vi "host.vi"() -> ()   [LabVIEW 2020]
uses:
  <vilib>/rvi/interface/RandomDataEmulation/nirviRandomDataOpen.vi
  <vilib>/rvi/interface/common/niFpgaCacheSessionInfoDynamic.vi
  <vilib>/Utility/error.llb/Error Cluster From Error Code.vi
  <vilib>/rvi/interface/common/niFpgaWaitOnOcc.vi
  <vilib>/rvi/errors/niLvFpgaAdjustHostInterfaceError.vi
  <vilib>/FPGAPlugInAG/Dynamic/niLvFpga_Run_Dynamic.vi
  <vilib>/FPGAPlugInAG/Dynamic/niLvFpga_Close_Dynamic.vi
  <vilib>/rvi/interface/nirviOpenFPGA/nirviOpenFPGA.xnode
  FFT.vi
  <vilib>/rvi/interface/nirviMethod/nirviMethod.xnode
  <vilib>/rvi/interface/nirviCloseFPGA/nirviCloseFPGA.xnode
  <vilib>/rvi/errors/niLvFpgaMergeErrorWithErrorCode.vi
  <vilib>/FPGAPlugInAG/Dynamic/niLvFpga_ReadFifo_Dynamic.vi
  <vilib>/Analysis/NI_AALPro.lvlib
  <vilib>/FPGAPlugInAG/Dynamic/niLvFpga_ConfigureFifo_Dynamic.vi
  <vilib>/FPGAPlugInAG/Dynamic/niLvFpga_StartFifo_Dynamic.vi
  <vilib>/FPGAPlugInAG/Dynamic/niLvFpga_WriteFifo_Dynamic.vi
panel:
  out "phase 2 index":dbl[](graph)
  out "phase 2 size":i32
  out "mag 2 index":dbl[](graph)
  out "mag 2 size":i32
  out "phase 2":fxp<+/-,32,15>[](array[numeric])
  out "mag 2":fxp<+/-,32,15>[](array[numeric])
  out "frequency index":dbl[](graph)
  out "frequency size":i32
  out "freq":fxp<+/-,32,15>[](array[numeric])
  out "magnitude":dbl[](graph)
  out "phase":dbl[](graph)
  out "phase size":i32
  out "mag size":i32
  out "phase":fxp<+/-,32,15>[](array[numeric])
  out "magnitude":fxp<+/-,32,15>[](array[numeric])
  out "Actual Depth":u32
  out "host to target":u32
  out "signal_target_to_host_fixed size(s)":i32
  out "target to host 1":u32
  out "signal target to host":dbl[][](graph)
  out "signal_target_to_host_fixed":fxp<+/-,24,7>[](array[numeric])
  out "Array 2":fxp<+/-,24,7>[](array[numeric])
  out "detrend acc":dbl[](graph)
  out "samples":i32
  out "input signal":T1(graph)
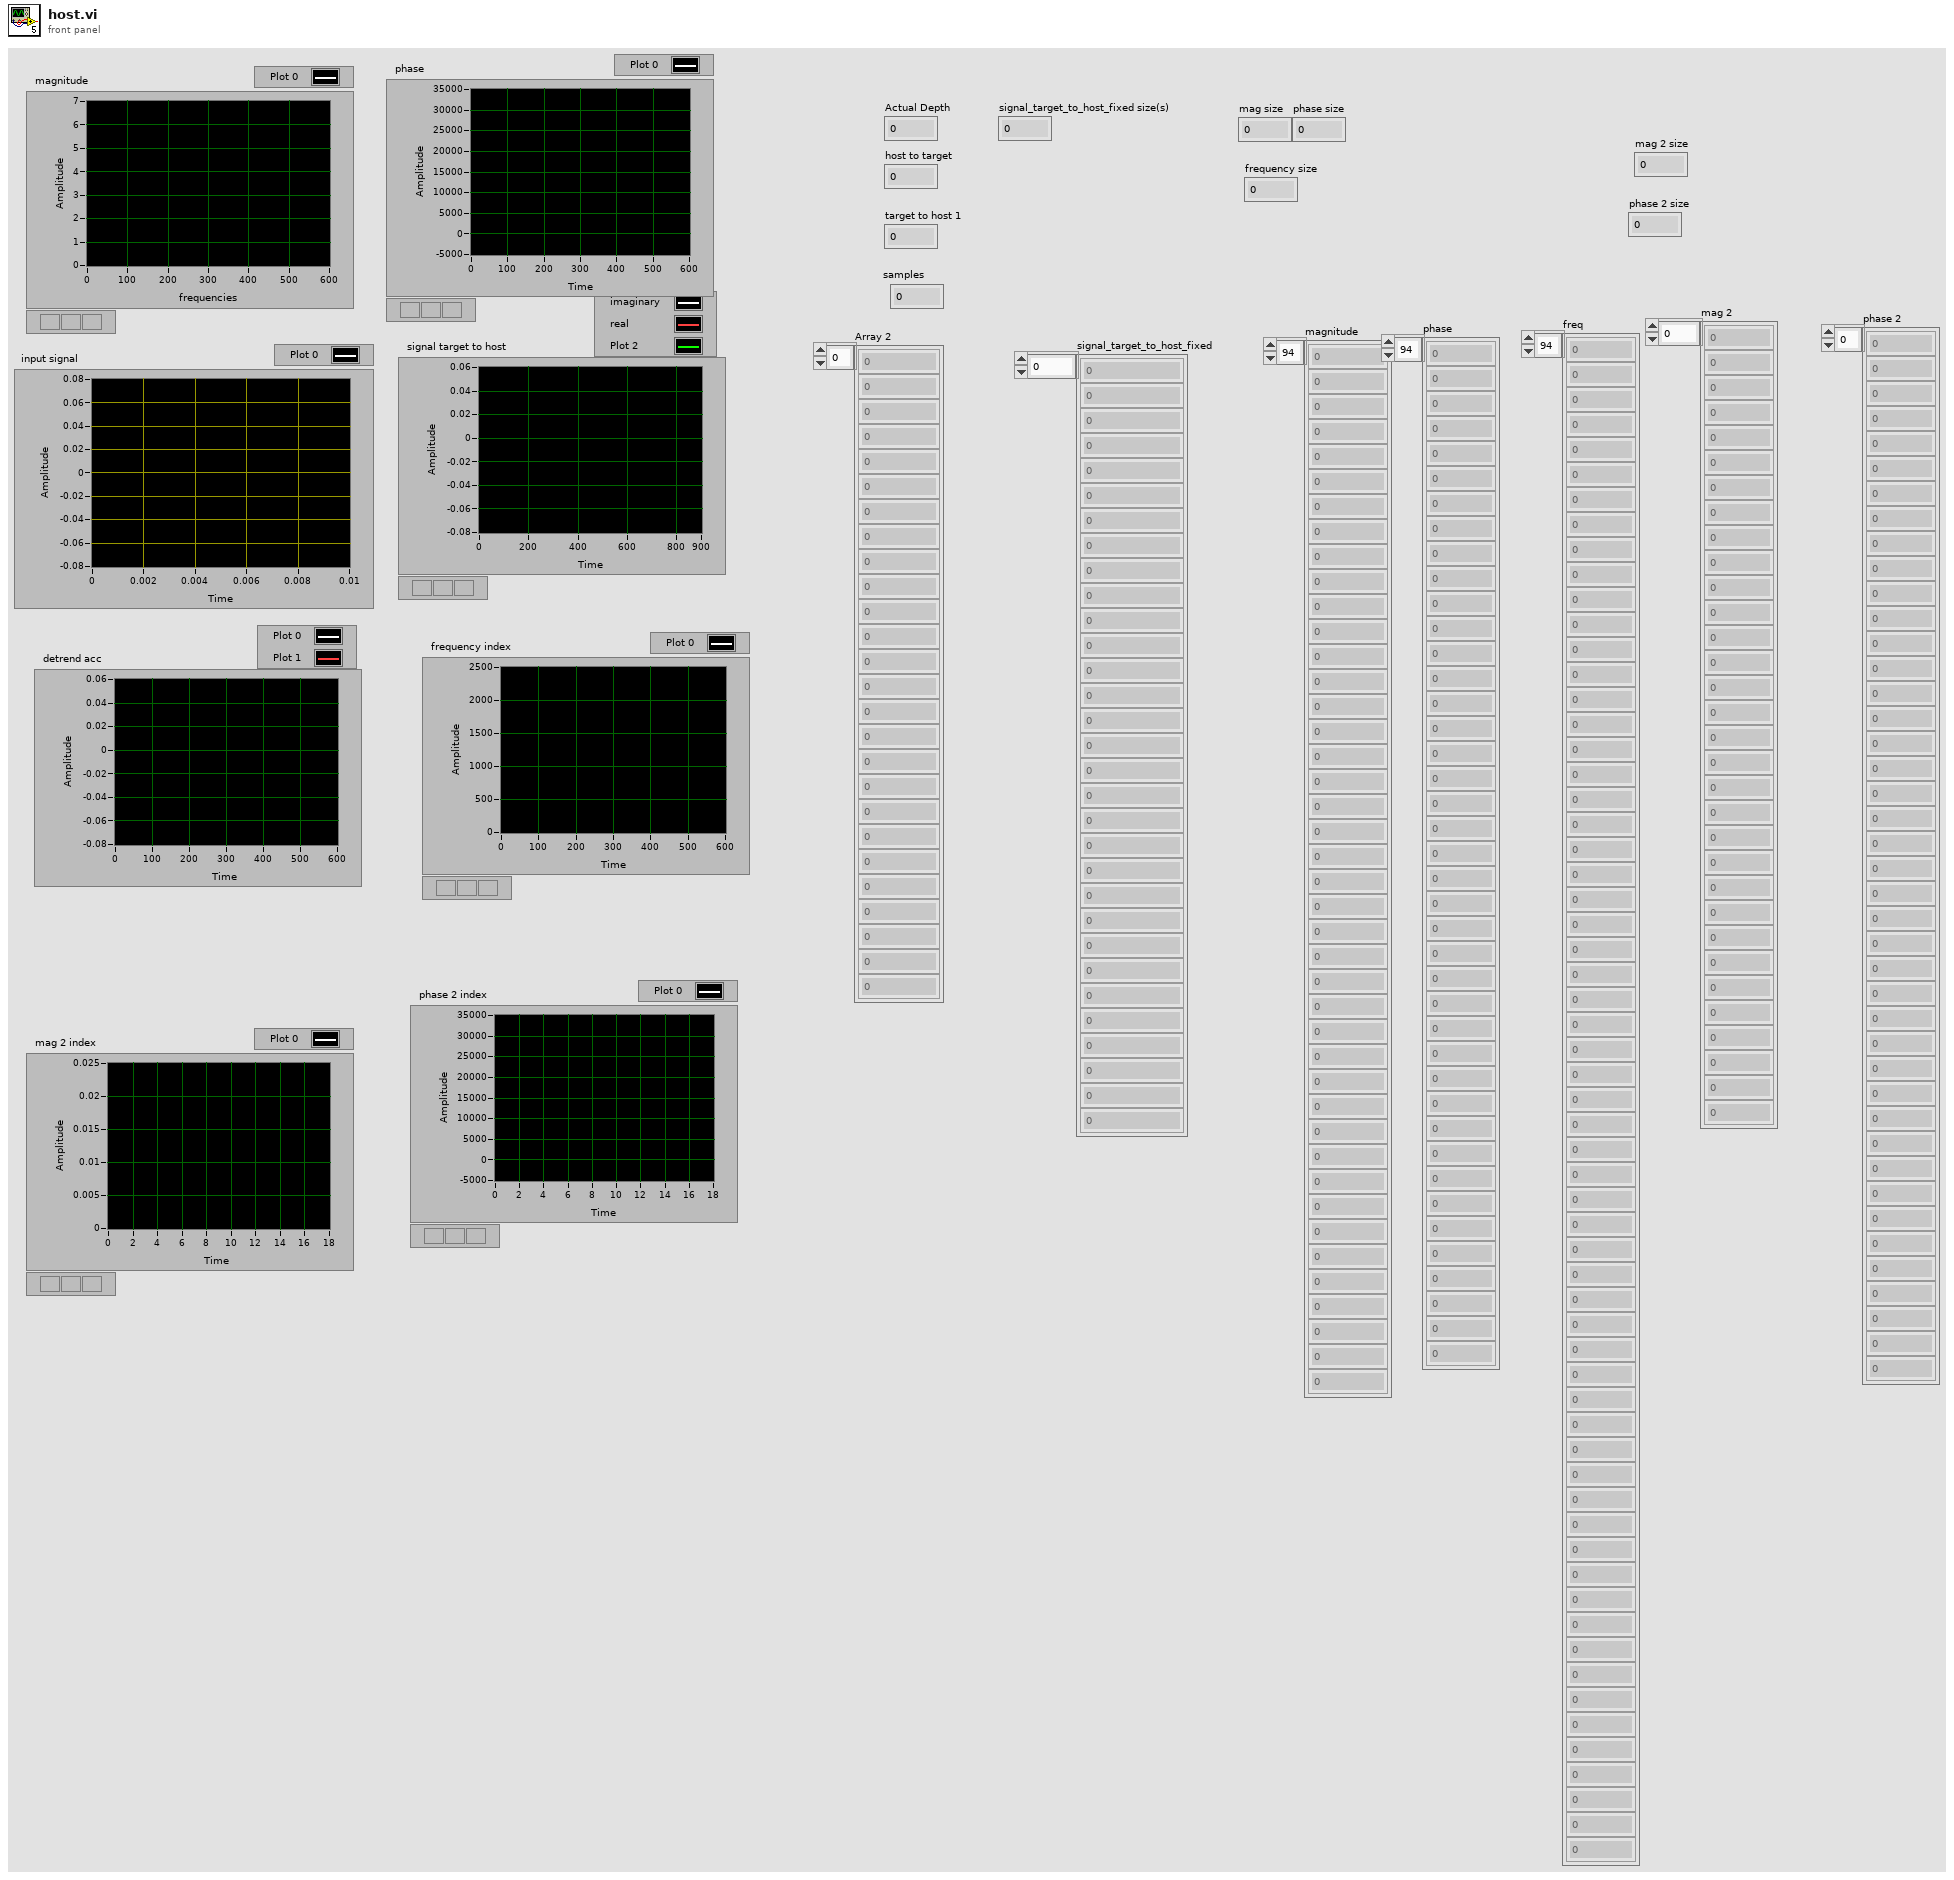
[diagram p1: front panel]
types:
  T1 = cluster{"array type (2D Dbl)":dbl[], "array type (2D Dbl)":dbl[]}
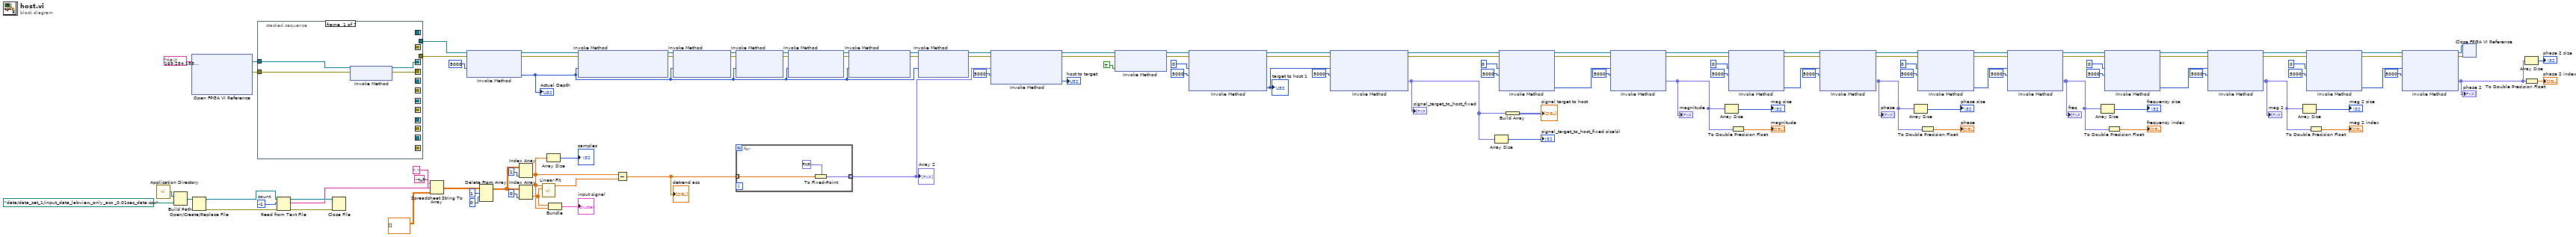
[diagram p0: block diagram]
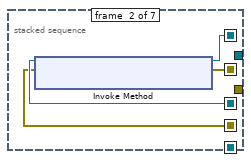
[diagram p2: hidden frame]
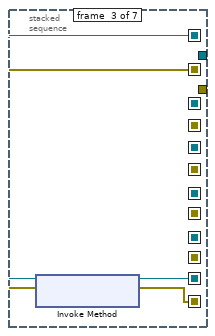
[diagram p3: hidden frame]
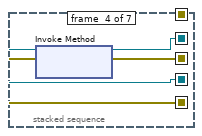
[diagram p4: hidden frame]
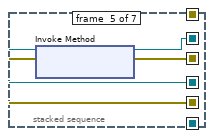
[diagram p5: hidden frame]
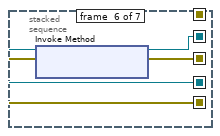
[diagram p6: hidden frame]
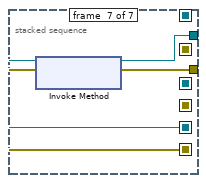
[diagram p7: hidden frame]
diagram:
  w110 = -1  # count
  n1 = call <vilib>:"Application Directory.vi"() -> ("Application Directory"=w114:path)
  n2 = Build Path(base path=w114, name or relative path=path "data/data_set_1/input_data_labview_only_acc _0.01sec_data.csv" ("default name")) -> (appended path=w113:path)
  n3 = xnode "Open FPGA VI Reference"("resource name"=tag "rio://169.254.183.73/RIO0") -> ("FPGA VI Reference Out"=w77:refnum<k20>, "error out"=w76:errorcluster)  [unwired: 1 in]
  n4 = Open/Create/Replace File(file path (use dialog)=w113) -> (refnum out=w118:refnum<file>, error out=w119:errorcluster)  [unwired: 5 in, 1 out]
  n5 = stacked-sequence {
    seq-local: [w121 _ _ _ _ _ _] -> [_ w127 _ _ _ _ _]
    seq-local: [w120 _ _ _ _ _ _] -> [_ w126 _ _ _ _ _]
    seq-local: [_ w125 _ _ _ _ _] -> [_ _ w131 _ _ _ _]
    seq-local: [_ w124 _ _ _ _ _] -> [_ _ w130 _ _ _ _]
    seq-local: [_ _ w129 _ _ _ _] -> [_ _ _ w135 _ _ _]
    seq-local: [_ _ w128 _ _ _ _] -> [_ _ _ w134 _ _ _]
    seq-local: [_ _ _ w133 _ _ _] -> [_ _ _ _ w139 _ _]
    seq-local: [_ _ _ w132 _ _ _] -> [_ _ _ _ w138 _ _]
    seq-local: [_ _ _ _ w137 _ _] -> [_ _ _ _ _ w143 _]
    seq-local: [_ _ _ _ w136 _ _] -> [_ _ _ _ _ w142 _]
    seq-local: [_ _ _ _ _ w141 _] -> [_ _ _ _ _ _ w147]
    seq-local: [_ _ _ _ _ w140 _] -> [_ _ _ _ _ _ w146]
    tunnel: w77 -> [w123 _ _ _ _ _ _]
    tunnel: w76 -> [w122 _ _ _ _ _ _]
    tunnel: [_ _ _ _ _ _ w145] -> w2
    tunnel: [_ _ _ _ _ _ w144] -> w1
    frame #0 {
      n6 = xnode "Invoke Method"("FPGA VI Reference In"=w123, "error in"=w122) -> ("FPGA VI Reference Out"=w121:refnum<k20>, "error out"=w120:errorcluster)
    }
    frame #1 {
      n7 = xnode "Invoke Method"("FPGA VI Reference In"=w127, "error in"=w126) -> ("FPGA VI Reference Out"=w125:refnum<k20>, "error out"=w124:errorcluster)
    }
    frame #2 {
      n8 = xnode "Invoke Method"("FPGA VI Reference In"=w131, "error in"=w130) -> ("FPGA VI Reference Out"=w129:refnum<k20>, "error out"=w128:errorcluster)
    }
    frame #3 {
      n9 = xnode "Invoke Method"("FPGA VI Reference In"=w135, "error in"=w134) -> ("FPGA VI Reference Out"=w133:refnum<k20>, "error out"=w132:errorcluster)
    }
    frame #4 {
      n10 = xnode "Invoke Method"("FPGA VI Reference In"=w139, "error in"=w138) -> ("FPGA VI Reference Out"=w137:refnum<k20>, "error out"=w136:errorcluster)
    }
    frame #5 {
      n11 = xnode "Invoke Method"("FPGA VI Reference In"=w143, "error in"=w142) -> ("FPGA VI Reference Out"=w141:refnum<k20>, "error out"=w140:errorcluster)
    }
    frame #6 {
      n12 = xnode "Invoke Method"("FPGA VI Reference In"=w147, "error in"=w146) -> ("FPGA VI Reference Out"=w144:refnum<k20>, "error out"=w145:errorcluster)
    }
  }
  n13 = Read from Text File(file (use dialog)=w118, count=w110, error in=w119) -> (refnum out=w117:refnum<file>, text=w115:string, error out=w116:errorcluster)  [unwired: 1 in, 1 out]
  n14 = Close File(refnum=w117, error in=w116) -> ()  [unwired: 2 out]
  n15 = Spreadsheet String To Array(delimiter (Tab)=",", format string="%f", spreadsheet string=w115, array type (2D Dbl)=dbl[][] []) -> (array=w107:dbl[][])
  n16 = xnode "Invoke Method"("FPGA VI Reference In"=w1, "error in"=w2, "Requested Depth"=u32 5000) -> ("FPGA VI Reference Out"=w75:refnum<k20>, "error out"=w74:errorcluster, "Actual Depth"=w11:u32)
  "Actual Depth" <- w11
  n17 = Delete From Array(array=w107, length=1, index (row)=0) -> (array with subset deleted=w102:dbl[][])  [unwired: 1 in, 1 out]
  n18 = Index Array(array=w102, index (col)=1 ("disabled index (col)")) -> (element=w92:dbl[])  [unwired: 1 in]
  n19 = Index Array(array=w102, index (col)=0 ("disabled index (col)")) -> (element=w94:dbl[])  [unwired: 1 in]
  n20 = call <vilib>:"Linear Fit.vi"("Y"=w92, "X"=w94) -> ("Best Linear Fit"=w93:dbl[])  [unwired: 9 in, 4 out]
  n21 = Array Size(array=w92) -> (size(s)=→"samples":i32)
  n22 = Bundle("array type (2D Dbl)"=w94, "array type (2D Dbl)"=w92) -> (→"input signal":T1)  [unwired: 1 in]
  n23 = xnode "Invoke Method"("FPGA VI Reference In"=w75, "error in"=w74, "Requested Depth"=w11) -> ("FPGA VI Reference Out"=w73:refnum<k20>, "error out"=w72:errorcluster)  [unwired: 1 out]
  n24 = Subtract(x=w92, y=w93) -> (x-y=w91:dbl[])
  "detrend acc" <- w91
  n25 = xnode "Invoke Method"("FPGA VI Reference In"=w73, "error in"=w72, "Requested Depth"=w11) -> ("FPGA VI Reference Out"=w71:refnum<k20>, "error out"=w70:errorcluster)  [unwired: 1 out]
  n26 = xnode "Invoke Method"("FPGA VI Reference In"=w71, "error in"=w70, "Requested Depth"=w11) -> ("FPGA VI Reference Out"=w37:refnum<k20>, "error out"=w36:errorcluster)  [unwired: 1 out]
  n27 = for {
    tunnel: [w149] -> w90 mode=indexing
    tunnel: w91 -> [w148] mode=indexing
    n28 = To Fixed-Point(fixed-point type=fxp<+/-,24,7> 0.0 ("f"), number=w148) -> (fixed-point=w149:fxp<+/-,24,7>)
  }
  "Array 2" <- w90
  n29 = xnode "Invoke Method"("FPGA VI Reference In"=w37, "error in"=w36, "Requested Depth"=w11) -> ("FPGA VI Reference Out"=w13:refnum<k20>, "error out"=w12:errorcluster)  [unwired: 1 out]
  n30 = xnode "Invoke Method"("FPGA VI Reference In"=w13, "error in"=w12, "Requested Depth"=w11) -> ("FPGA VI Reference Out"=w15:refnum<k20>, "error out"=w14:errorcluster)  [unwired: 1 out]
  n31 = xnode "Invoke Method"("FPGA VI Reference In"=w15, "error in"=w14, "Requested Depth"=w11) -> ("FPGA VI Reference Out"=w4:refnum<k20>, "error out"=w3:errorcluster)  [unwired: 1 out]
  n32 = xnode "Invoke Method"("FPGA VI Reference In"=w4, "error in"=w3, "Data"=w90, "Timeout (ms)"=5000) -> ("FPGA VI Reference Out"=w99:refnum<k20>, "error out"=w98:errorcluster, "Empty Elements Remaining"=→"host to target":u32)
  n33 = xnode "Invoke Method"("FPGA VI Reference In"=w99, "error in"=w98, "Wait Until Done (F)"=TRUE) -> ("FPGA VI Reference Out"=w81:refnum<k20>, "error out"=w80:errorcluster)
  n34 = xnode "Invoke Method"("FPGA VI Reference In"=w81, "error in"=w80, "Number of Elements"=u32 0, "Timeout (ms)"=5000) -> ("FPGA VI Reference Out"=w89:refnum<k20>, "error out"=w88:errorcluster, "Elements Remaining"=w87:u32)  [unwired: 1 out]
  "target to host 1" <- w87
  n35 = xnode "Invoke Method"("FPGA VI Reference In"=w89, "error in"=w88, "Number of Elements"=w87, "Timeout (ms)"=5000) -> ("FPGA VI Reference Out"=w52:refnum<k20>, "error out"=w51:errorcluster, "Data"=w83:fxp<+/-,24,7>[])  [unwired: 1 out]
  "signal_target_to_host_fixed" <- w83
  n36 = Array Size(array=w83) -> (size(s)=→"signal_target_to_host_fixed size(s)":i32)
  n37 = xnode "Invoke Method"("FPGA VI Reference In"=w52, "error in"=w51, "Number of Elements"=u32 0, "Timeout (ms)"=5000) -> ("FPGA VI Reference Out"=w66:refnum<k20>, "error out"=w65:errorcluster, "Elements Remaining"=w60:u32)  [unwired: 1 out]
  n38 = Build Array(w83) -> (→"signal target to host":fxp<+/-,24,7>[][])
  n39 = xnode "Invoke Method"("FPGA VI Reference In"=w66, "error in"=w65, "Number of Elements"=w60, "Timeout (ms)"=5000) -> ("FPGA VI Reference Out"=w64:refnum<k20>, "error out"=w63:errorcluster, "Data"=w50:fxp<+/-,32,16>[])  [unwired: 1 out]
  "magnitude" <- w50
  n40 = Array Size(array=w50) -> (size(s)=→"mag size":i32)
  n41 = xnode "Invoke Method"("FPGA VI Reference In"=w64, "error in"=w63, "Number of Elements"=u32 0, "Timeout (ms)"=5000) -> ("FPGA VI Reference Out"=w62:refnum<k20>, "error out"=w61:errorcluster, "Elements Remaining"=w56:u32)  [unwired: 1 out]
  n42 = To Double Precision Float(number=w50) -> (double precision float=→"magnitude":dbl[])
  n43 = xnode "Invoke Method"("FPGA VI Reference In"=w62, "error in"=w61, "Number of Elements"=w56, "Timeout (ms)"=5000) -> ("FPGA VI Reference Out"=w39:refnum<k20>, "error out"=w38:errorcluster, "Data"=w49:fxp<+/-,32,16>[])  [unwired: 1 out]
  "phase" <- w49
  n44 = Array Size(array=w49) -> (size(s)=→"phase size":i32)
  n45 = xnode "Invoke Method"("FPGA VI Reference In"=w39, "error in"=w38, "Number of Elements"=u32 0, "Timeout (ms)"=5000) -> ("FPGA VI Reference Out"=w48:refnum<k20>, "error out"=w47:errorcluster, "Elements Remaining"=w44:u32)  [unwired: 1 out]
  n46 = To Double Precision Float(number=w49) -> (double precision float=→"phase":dbl[])
  n47 = xnode "Invoke Method"("FPGA VI Reference In"=w48, "error in"=w47, "Number of Elements"=w44, "Timeout (ms)"=5000) -> ("FPGA VI Reference Out"=w23:refnum<k20>, "error out"=w22:errorcluster, "Data"=w41:fxp<+/-,32,16>[])  [unwired: 1 out]
  "freq" <- w41
  n48 = Array Size(array=w41) -> (size(s)=→"frequency size":i32)
  n49 = xnode "Invoke Method"("FPGA VI Reference In"=w23, "error in"=w22, "Number of Elements"=u32 0, "Timeout (ms)"=5000) -> ("FPGA VI Reference Out"=w35:refnum<k20>, "error out"=w34:errorcluster, "Elements Remaining"=w31:u32)  [unwired: 1 out]
  n50 = To Double Precision Float(number=w41) -> (double precision float=→"frequency index":dbl[])
  n51 = xnode "Invoke Method"("FPGA VI Reference In"=w35, "error in"=w34, "Number of Elements"=w31, "Timeout (ms)"=5000) -> ("FPGA VI Reference Out"=w21:refnum<k20>, "error out"=w20:errorcluster, "Data"=w17:fxp<+/-,32,16>[])  [unwired: 1 out]
  "mag 2" <- w17
  n52 = Array Size(array=w17) -> (size(s)=→"mag 2 size":i32)
  n53 = xnode "Invoke Method"("FPGA VI Reference In"=w21, "error in"=w20, "Number of Elements"=u32 0, "Timeout (ms)"=5000) -> ("FPGA VI Reference Out"=w29:refnum<k20>, "error out"=w28:errorcluster, "Elements Remaining"=w25:u32)  [unwired: 1 out]
  n54 = To Double Precision Float(number=w17) -> (double precision float=→"mag 2 index":dbl[])
  n55 = xnode "Invoke Method"("FPGA VI Reference In"=w29, "error in"=w28, "Number of Elements"=w25, "Timeout (ms)"=5000) -> ("FPGA VI Reference Out"=w6:refnum<k20>, "error out"=w5:errorcluster, "Data"=w16:fxp<+/-,32,16>[])  [unwired: 1 out]
  "phase 2" <- w16
  n56 = xnode "Close FPGA VI Reference"("FPGA VI Reference In"=w6, "error in"=w5) -> ()  [unwired: 1 out]
  n57 = Array Size(array=w16) -> (size(s)=→"phase 2 size":i32)
  n58 = To Double Precision Float(number=w16) -> (double precision float=→"phase 2 index":dbl[])
